vi "Find IntelliSense Control.vi"(9 "IntelliSenseStringControl":refnum<class "IntelliSenseStringControl.lvclass">, 11 "IntelliSense String []":refnum<class "IntelliSenseStringControl.lvclass">[](array[class])) -> (0 "Found?":bool, 1 "Found IntelliSenseStringControl":refnum<class "IntelliSenseStringControl.lvclass">, 3 "Other IntelliSense String []":refnum<class "IntelliSenseStringControl.lvclass">[](array[class]))   [LabVIEW 2016, in "StringIntelliSense.lvlib" / "IntelliSenseStringControl.lvclass"]
uses:
  IntelliSenseStringControl.lvclass
  IntelliSenseStringControl.lvclass/IntelliSenseStringControl.ctl
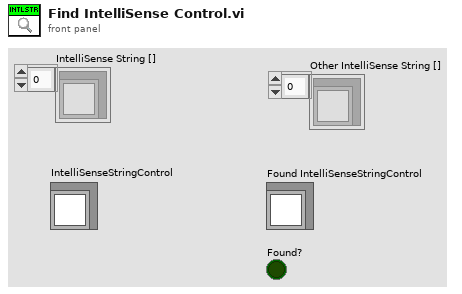
[diagram p1: front panel]
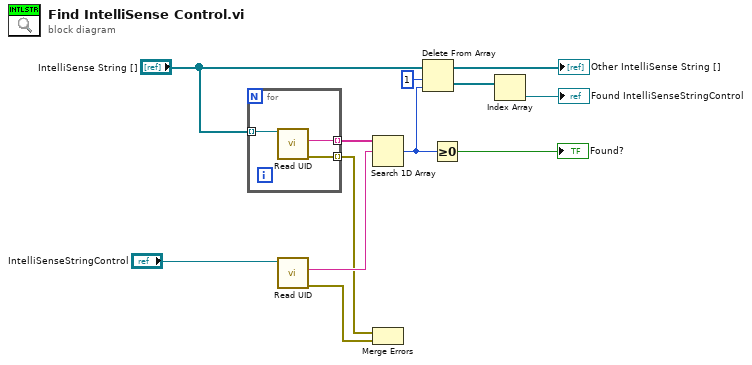
[diagram p0: block diagram]
diagram:
  n1 = for {
    tunnel: "IntelliSense String []" -> [w15] mode=indexing
    tunnel: [w14] -> w12 mode=indexing
    tunnel: [w13] -> w5 mode=indexing
    n2 = call "Read UID.vi"("IntelliSenseStringControl in"=w15) -> ("error out"=w13:errorcluster, "UID"=w14:string)  [unwired: 8 in, 1 out]
  }
  n3 = call "Read UID.vi"("IntelliSenseStringControl in"="IntelliSenseStringControl") -> ("error out"=w4:errorcluster, "UID"=w11:string)  [unwired: 8 in, 1 out]
  n4 = Search 1D Array(1D array=w12, element=w11) -> (index of element=w8:i32)  [unwired: 1 in]
  n5 = Merge Errors(w5, w4) -> ()  [unwired: 1 out]
  n6 = Delete From Array(array="IntelliSense String []", length=1, index=w8) -> (deleted portion=w9:refnum<class "IntelliSenseStringControl.lvclass">[], array with subset deleted=→"Other IntelliSense String []":refnum<class "IntelliSenseStringControl.lvclass">[])
  n7 = Greater Or Equal To 0?(x=w8) -> (x >= 0?=→"Found?":bool)
  n8 = Index Array(array=w9) -> (element=→"Found IntelliSenseStringControl":refnum<class "IntelliSenseStringControl.lvclass">)  [unwired: 1 in]
